vi "Keithley 6514 Current Config.vi"(0 "Resource In":refnum<visa-resource-name>, 1 "Check For SCPI Errors? (T)":bool=TRUE, 5 "NPLC value (1.0)":dbl=1.0 min=0.01 max=10.0 step=0.01 format="%.2f", 7 "range (autorange:0)":u16(ring) items=["autorange", "set min range", "set max range", "set range value"], 9 "range value (A) (210e-6)":dbl=0.0002099999983329326 min=0.0 max=0.020999999716877937 step=9.999999960041972e-12 format="%^.2e", 11 "error in (no error)":T1, 12 "Autorange Upper Limit (A) (21e-3)":dbl=0.020999999716877937 min=0.0 max=0.020999999716877937 step=9.999999960041972e-12 format="%^.2e", 13 "Autorange Lower Limit (A) (21e-12)":dbl=2.100000034976901e-11 min=0.0 max=0.020999999716877937 step=9.999999960041972e-12 format="%^.2e", 14 "Damping (OFF:F)":bool) -> (4 "Resource Out (dupl)":refnum<visa-resource-name>, 15 "error out":T1)   [LabVIEW 2014, in "KE6514Driver.lvlib"]
doc: "This VI is used to configure the settings for current measurements.\n\nNPLC:\n0.01 to 10\n\nDamping:\nTRUE = on\nFALSE = Off\n\nRange:\n0 = Autoranging\n1 = Set minimum range\n2 = Set maximum range\n3 = Set range by value\n\nRange value:\n0 to 2.1e-2\n\nAutorange Upper Limit:\n0 to 2.1e-2 (2.1e-2 default)\n\nAutorange Lower Limit:\n0 to 2.1e-2 (2.1e-11 default)"
uses:
  KE6514Driver.lvlib
panel:
  # "on\noff"
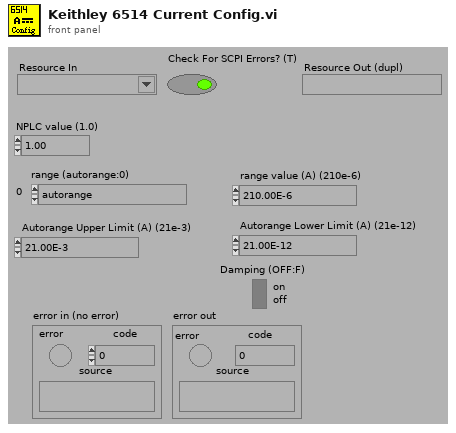
[diagram p1: front panel]
types:
  T1 = cluster{"error":bool, "code":i32, "source":string}
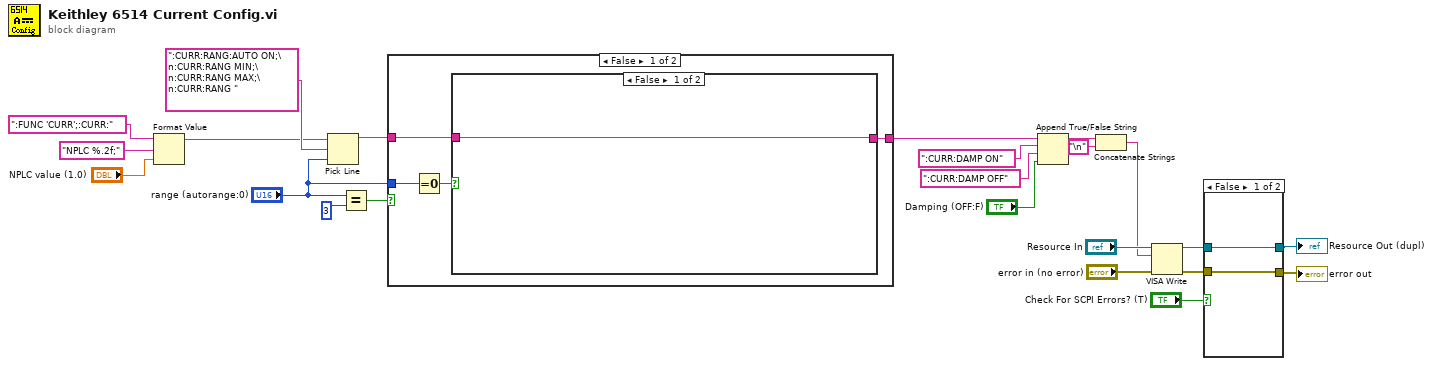
[diagram p0: block diagram]
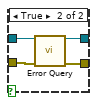
[diagram p2: hidden frame]
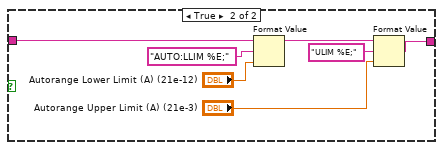
[diagram p3: hidden frame]
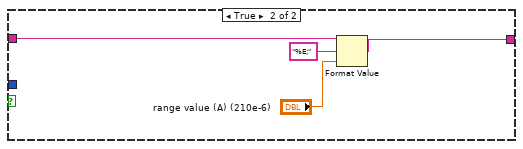
[diagram p4: hidden frame]
diagram:
  n1 = Format Value(string ("")=":FUNC 'CURR';:CURR:", format string="NPLC %.2f;", value (0)="NPLC value (1.0)") -> (output string=w13:string)
  n2 = Pick Line(string ("")=w13, multi-line string=":CURR:RANG:AUTO ON;\n:CURR:RANG MIN;\n:CURR:RANG MAX;\n:CURR:RANG ", line index="range (autorange:0)") -> (output string=w23:string)
  n3 = Equal?(x="range (autorange:0)", y=u16 3) -> (x = y?=w22:bool)
  n4 = case shown="False" w22 {
    tunnel: w23 -> [w25 w37]
    tunnel: [w24 w36] -> w11
    tunnel: "range (autorange:0)" -> [w27 _]
    frame False {
      n5 = Equal To 0?(x=w27) -> (x = 0?=w26:bool)
      n6 = case shown="False" w26 {
        tunnel: w25 -> [w28 w34]
        tunnel: [w28 w29] -> w24
        frame False {
        }
        frame True {
          n7 = Format Value(string ("")=w34, format string="AUTO:LLIM %E;", value (0)="Autorange Lower Limit (A) (21e-12)") -> (output string=w32:string)
          n8 = Format Value(string ("")=w32, format string="ULIM %E;", value (0)="Autorange Upper Limit (A) (21e-3)") -> (output string=w29:string)
        }
      }
    }
    frame True {
      n9 = Format Value(string ("")=w37, format string="%E;", value (0)="range value (A) (210e-6)") -> (output string=w36:string)
    }
  }
  n10 = Append True/False String(1:"Damping (OFF:F)", 2:":CURR:DAMP OFF", 3:":CURR:DAMP ON", 4:w11) -> (0:w9:string)
  n11 = Concatenate Strings(w9, "\n") -> (w7:string)
  n12 = VISA Write(VISA resource name="Resource In", write buffer=w7, error in (no error)="error in (no error)") -> (VISA resource name out=w4:refnum<visa-resource-name>, error out=w3:errorcluster)  [unwired: 1 out]
  n13 = case shown="False" "Check For SCPI Errors? (T)" {
    tunnel: w4 -> [w41 w45]
    tunnel: w3 -> [w40 w44]
    tunnel: [w41 w43] -> w1
    tunnel: [w40 w42] -> w2
    frame False {
    }
    frame True {
      n14 = call "Error Query.vi"("VISA Resource In"=w45, "error in (no error)"=w44) -> ("VISA Resource Out (dupl)"=w43:refnum<visa-resource-name>, "error out"=w42:errorcluster)  [unwired: 10 in, 2 out]
    }
  }
  "error out" <- w2
  "Resource Out (dupl)" <- w1
